vi "SVM Train C_SVC.vi"(7 "Options":T9={"cache_size"=200.0, "eps"=0.001, "shrinking"=TRUE, "probability"=FALSE}, 8 "error in (no error)":errorcluster, 9 "Param C_SVC":T1={"C"=1.0, "weight_label"=[], "weight"=[]}, 10 "Kernel":T8, 11 "Problem":T7) -> (0 "error out":errorcluster, 3 "Model":T2)   [LabVIEW 2014]
doc: "This function constructs and returns an SVM model according to the given training data and parameters."
uses:
  Controls/Options Training.ctl
  Controls/Kernel.ctl
  Wrapper API/Controls/svm_kernel_type.ctl
  Wrapper API/Controls/svm_problem.ctl
  Wrapper API/Controls/svm_node.ctl
  Wrapper API/Controls/svm_model.ctl
  Wrapper API/Controls/svm_parameter.ctl
  Wrapper API/Controls/svm_type.ctl
  Controls/Parameters C_SVC.ctl
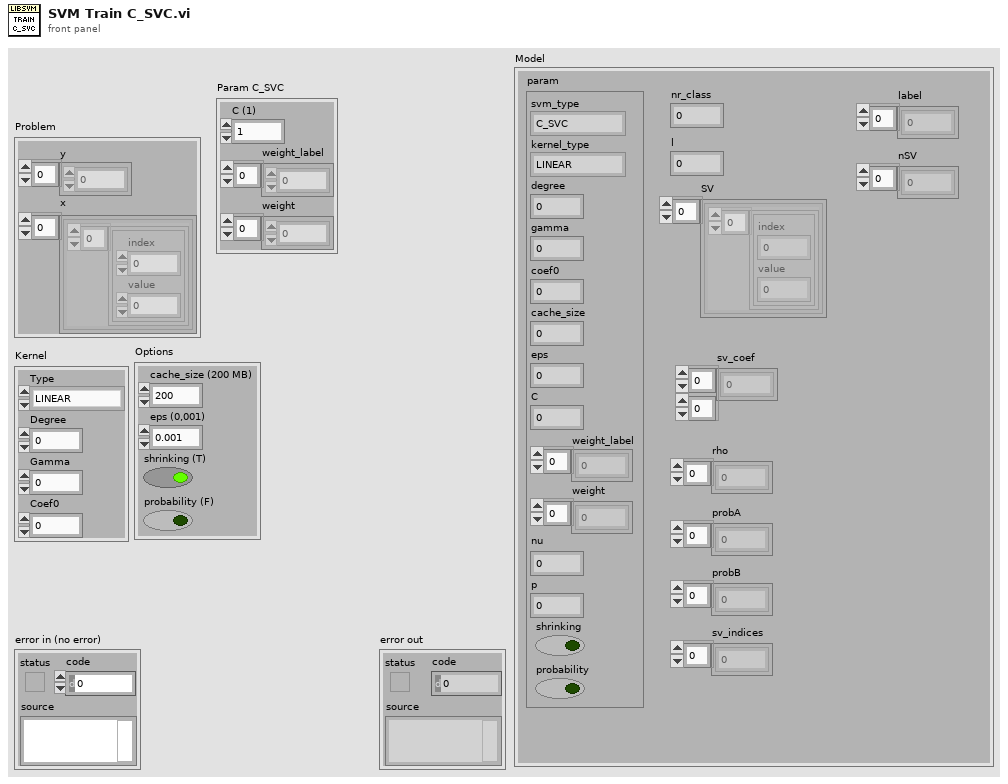
[diagram p1: front panel]
types:
  T1 = typedef "Parameters C_SVC.ctl" = cluster{"C":dbl, "weight_label":i32[], "weight":dbl[]}
  T2 = typedef "svm_model.ctl" = cluster{"param":T3, "nr_class":i32, "l":i32, "SV":cluster{"Array":T6[]}[], "sv_coef":dbl[][], "rho":dbl[], "probA":dbl[], "probB":dbl[], "sv_indices":i32[], "label":i32[], "nSV":i32[]}
  T3 = typedef "svm_parameter.ctl" = cluster{"svm_type":T4, "kernel_type":T5, "degree":i32, "gamma":dbl, "coef0":dbl, "cache_size":dbl, "eps":dbl, "C":dbl, "weight_label":i32[], "weight":dbl[], "nu":dbl, "p":dbl, "shrinking":bool, "probability":bool}
  T4 = typedef "svm_type.ctl" = enum32{"C_SVC", "NU_SVC", "ONE_CLASS", "EPSILON_SVR", "NU_SVR"}
  T5 = typedef "svm_kernel_type.ctl" = enum32{"LINEAR", "POLY", "RBF", "SIGMOID", "PRECOMPUTED"}
  T6 = typedef "svm_node.ctl" = cluster{"index":i32, "value":dbl}
  T7 = typedef "svm_problem.ctl" = cluster{"y":dbl[], "x":cluster{T6[]}[]}
  T8 = typedef "Kernel.ctl" = cluster{"Type":T5, "Degree":i32, "Gamma":dbl, "Coef0":dbl}
  T9 = typedef "Options Training.ctl" = cluster{"cache_size":dbl, "eps":dbl, "shrinking":bool, "probability":bool}
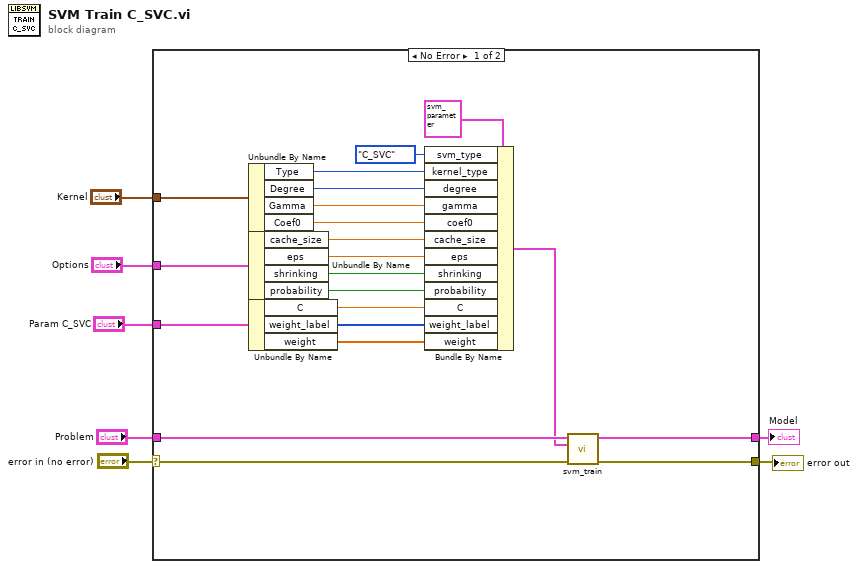
[diagram p0: block diagram]
diagram:
  n1 = case shown="No Error" "error in (no error)" {
    selector: "error in (no error)" -> [w28 w29]
    tunnel: [w27 w29] -> w7
    tunnel: "Problem" -> [w25 _]
    tunnel: "Kernel" -> [w24 _]
    tunnel: [w17 _] -> w3
    tunnel: "Options" -> [w13 _]
    tunnel: "Param C_SVC" -> [w14 _]
    frame No Error {
      n2 = Unbundle By Name(w24) -> ("Type"=w23:T5, "Degree"=w22:i32, "Gamma"=w21:dbl, "Coef0"=w20:dbl)
      n3 = Unbundle By Name(w13) -> ("cache_size"=w16:dbl, "eps"=w15:dbl, "shrinking"=w12:bool, "probability"=w11:bool)
      n4 = Unbundle By Name(w14) -> ("C"=w10:dbl, "weight_label"=w9:i32[], "weight"=w8:dbl[])
      n5 = Bundle By Name(cluster=T3 {"svm_type"=enum."C_SVC", "kernel_type"=enum."LINEAR", "degree"=0, "gamma"=0.0, "coef0"=0.0, "cache_size"=0.0, "eps"=0.0, "C"=0.0, "weight_label"=[], "weight"=[], "nu"=0.0, "p"=0.0, "shrinking"=FALSE, "probability"=FALSE} ("svm_parameter"), "svm_type"=svm_type."C_SVC", "kernel_type"=w23, "degree"=w22, "gamma"=w21, "coef0"=w20, "cache_size"=w16, "eps"=w15, "shrinking"=w12, "probability"=w11, "C"=w10, "weight_label"=w9, "weight"=w8) -> (w18:T3)
      n6 = call "svm_train.vi"("error in (no error)"=w28, "Parameters"=w18, "Problem"=w25) -> ("error out"=w27:errorcluster, "Model"=w17:T2)  [unwired: 7 in]
    }
    frame Error {
    }
  }
  "error out" <- w7
  "Model" <- w3
